vi "error log fg.vi"(2 "Error":string, 3 "Log Mode":enum16{"Get", "Set", "Clear"}(ring)) -> (0 "Errors":string, 1 "Errors Present":bool)   [LabVIEW 2013]
panel:
  # "Error Logging FG"
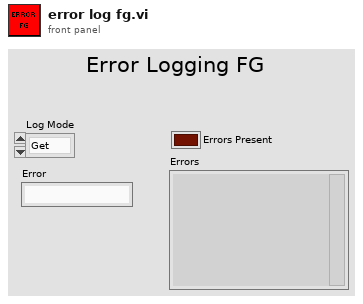
[diagram p1: front panel]
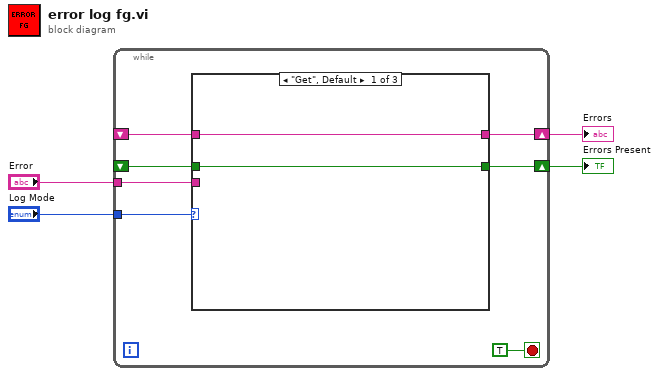
[diagram p0: block diagram]
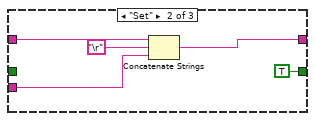
[diagram p2: hidden frame]
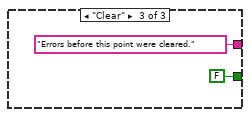
[diagram p3: hidden frame]
diagram:
  n1 = while {
    tunnel: "Error" -> [w9]
    shift-right: [w10] -> w2
    shift-left: _ -> [w8]
    tunnel: "Log Mode" -> [w11]
    shift-right: [w6] -> w1
    shift-left: _ -> [w5]
    stop <- TRUE stop-if-true
    n2 = case shown="\"Get\", Default" w11 {
      tunnel: [w13 w18 "Errors before this point were cleared."] -> w10
      tunnel: w9 -> [_ w15 _]
      tunnel: w8 -> [w13 w17 _]
      tunnel: [w12 TRUE FALSE] -> w6
      tunnel: w5 -> [w12 _ _]
      frame "Get", Default {
      }
      frame "Set" {
        n3 = Concatenate Strings(w17, "\r", w15) -> (w18:string)
      }
      frame "Clear" {
      }
    }
  }
  "Errors" <- w2
  "Errors Present" <- w1
